vi "Check_Lid_Position.vi"(8 "error in (no error)":errorcluster, 11 "Device":string) -> (0 "error out":errorcluster, 2 "data":bool)   [LabVIEW 2015]
uses:
  <vilib>/DAQmx/read.llb/DAQmx Read (Digital Bool 1Line 1Point).vi
  <vilib>/DAQmx/create/channels.llb/DAQmx Create Channel (DI-Digital Input).vi
  <vilib>/DAQmx/miscellaneous.llb/DAQmx Fill In Error Info.vi
panel:
  # "\"Dev5/port1/line0\""
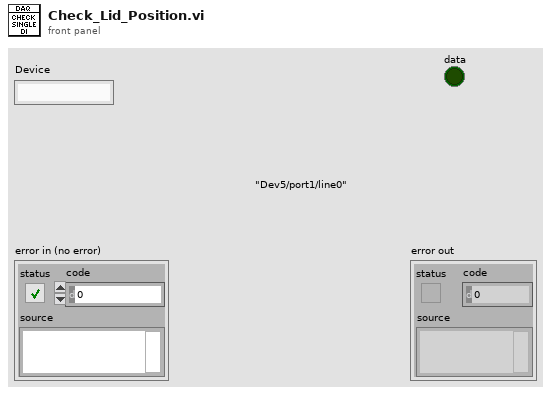
[diagram p1: front panel]
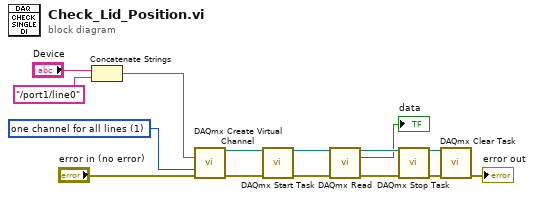
[diagram p0: block diagram]
diagram:
  w15 = 1 items=["one channel for each line", "one channel for all lines"] ("line grouping")
  n1 = Concatenate Strings("Device", "/port1/line0" ("string")) -> (w2:string)
  n2 = call-poly <vilib>:"DAQmx Create Virtual Channel.vi"("lines"=w2, "line grouping"=w15, "error in"="error in (no error)") -> ("task out"=w14:refnum<k21>, "error out"=w13:errorcluster)  [unwired: 11 in]
  n3 = call <vilib>:"DAQmx Start Task.vi"("task/channels in"=w14, "error in"=w13) -> ("task out"=w12:refnum<k21>, "error out"=w11:errorcluster)  [unwired: 12 in]
  n4 = call-poly <vilib>:"DAQmx Read.vi"("task/channels in"=w12, "error in"=w11) -> ("task out"=w10:refnum<k21>, "data"=→"data":bool, "error out"=w9:errorcluster)  [unwired: 11 in]
  n5 = call <vilib>:"DAQmx Stop Task.vi"("task/channels in"=w10, "error in"=w9) -> ("task out"=w8:refnum<k21>, "error out"=w7:errorcluster)  [unwired: 12 in]
  n6 = call <vilib>:"DAQmx Clear Task.vi"("task in"=w8, "error in"=w7) -> ("error out"=→"error out":errorcluster)  [unwired: 13 in]
